vi "压力量程转换为工程量.vi"(2 "量程":i32, 3 "数值输入":i32) -> (1 "数值输出":dbl)   [LabVIEW 2014]
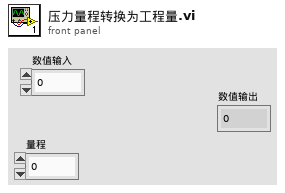
[diagram p1: front panel]
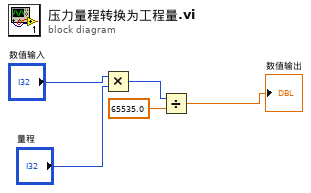
[diagram p0: block diagram]
diagram:
  n1 = Multiply(x="数值输入", y="量程") -> (x*y=w3:i32)
  n2 = Divide(x=w3, y=65535.0) -> (x/y=→"数值输出":dbl)
